vi "Testing Run.vi"(1 "FrequencyCounter":refnum<visa-resource-name>, 2 "connection information":path, 4 "Output Powers":bool, 5 "Warmup":bool, 6 "PHN Test":bool, 7 "System Number":string, 8 "error in":errorcluster, 9 "Osc Test":bool, 10 "FVT Test":bool, 11 "Arduino":refnum<visa-resource-name>) -> (0 "error out":errorcluster, 3 "Arduino out":refnum<visa-resource-name>)   [LabVIEW 2024]
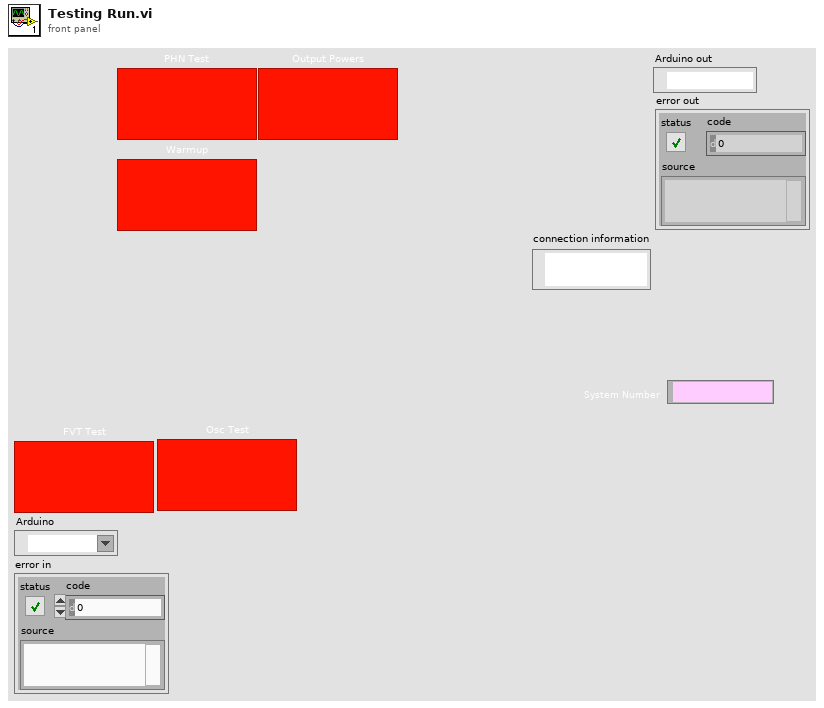
[diagram p1: front panel]
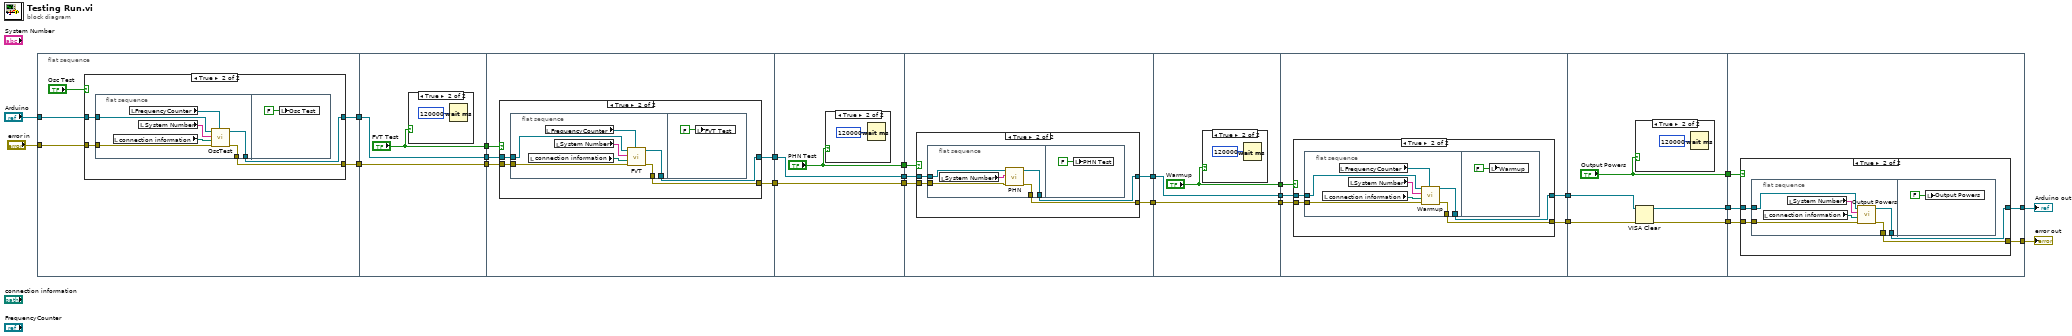
[diagram p0: block diagram]
diagram:
  n1 = flat-sequence {
    tunnel: [w26] -> w8
    tunnel: [w25] -> w6
    tunnel: "error in" -> [w28]
    tunnel: "Arduino" -> [w27]
    tunnel: w8 -> [w46]
    tunnel: [w46] -> w7
    tunnel: w6 -> [w45]
    tunnel: [w45] -> w5
    tunnel: ["FVT Test"] -> w4
    tunnel: w7 -> [w52]
    tunnel: w5 -> [w51]
    tunnel: [w50] -> w12
    tunnel: [w49] -> w10
    tunnel: w4 -> [w48]
    tunnel: w12 -> [w69]
    tunnel: [w69] -> w11
    tunnel: w10 -> [w68]
    tunnel: [w68] -> w9
    tunnel: ["PHN Test"] -> w3
    tunnel: w11 -> [w75]
    tunnel: w9 -> [w74]
    tunnel: [w73] -> w16
    tunnel: [w72] -> w14
    tunnel: w3 -> [w71]
    tunnel: w16 -> [w90]
    tunnel: [w90] -> w15
    tunnel: w14 -> [w89]
    tunnel: [w89] -> w13
    tunnel: ["Warmup"] -> w2
    tunnel: w15 -> [w96]
    tunnel: w13 -> [w94]
    tunnel: [w95] -> w20
    tunnel: [w93] -> w18
    tunnel: w2 -> [w92]
    tunnel: w20 -> [w115]
    tunnel: [w112] -> w19
    tunnel: w18 -> [w114]
    tunnel: [w113] -> w17
    tunnel: ["Output Powers"] -> w1
    tunnel: [w118] -> w21
    tunnel: [w120] -> w22
    tunnel: w19 -> [w121]
    tunnel: w17 -> [w119]
    tunnel: w1 -> [w117]
    frame #0 {
      n2 = case shown="True" "Osc Test" {
        tunnel: w28 -> [w30 w35]
        tunnel: w27 -> [w31 w34]
        tunnel: [w31 w33] -> w26
        tunnel: [w30 w32] -> w25
        frame False {
        }
        frame True {
          n3 = flat-sequence {
            tunnel: w35 -> [w41]
            tunnel: w34 -> [w40]
            tunnel: [w39] -> w33
            tunnel: [w38] -> w32
            frame #0 {
              n4 = local read "connection information"() -> (w37:path)
              n5 = local read "FrequencyCounter"() -> (w36:refnum<visa-resource-name>)
              n6 = local read "System Number"() -> (w42:string)
              n7 = call "OscTest.vi"("FrequencyCounter"=w36, "error in"=w41, "connection information"=w37, "System Number"=w42, "Arduino"=w40) -> ("error out"=w38:errorcluster, "Arduino out"=w39:refnum<visa-resource-name>)  [unwired: 5 in]
            }
            frame #1 {
              n8 = local write "Osc Test"(FALSE ("Osc Test")) -> ()
            }
          }
        }
      }
    }
    frame #1 {
      n9 = case shown="True" "FVT Test" {
        frame False {
        }
        frame True {
          n10 = Wait (ms)(milliseconds to wait=u32 120000) -> ()  [unwired: 1 out]
        }
      }
    }
    frame #2 {
      n11 = case shown="True" w48 {
        tunnel: w51 -> [w54 w57]
        tunnel: w52 -> [w53 w58]
        tunnel: [w53 w56] -> w50
        tunnel: [w54 w55] -> w49
        frame False {
        }
        frame True {
          n12 = flat-sequence {
            tunnel: w58 -> [w65]
            tunnel: w57 -> [w64]
            tunnel: [w62] -> w56
            tunnel: [w61] -> w55
            frame #0 {
              n13 = local read "connection information"() -> (w60:path)
              n14 = local read "FrequencyCounter"() -> (w59:refnum<visa-resource-name>)
              n15 = local read "System Number"() -> (w63:string)
              n16 = call "FVT.vi"("FrequencyCounter"=w59, "error in"=w64, "connection information"=w60, "System Number"=w63, "Arduino"=w65) -> ("error out"=w61:errorcluster, "Arduino out"=w62:refnum<visa-resource-name>)  [unwired: 5 in]
            }
            frame #1 {
              n17 = local write "FVT Test"(FALSE ("FVT Test")) -> ()
            }
          }
        }
      }
    }
    frame #3 {
      n18 = case shown="True" "PHN Test" {
        frame False {
        }
        frame True {
          n19 = Wait (ms)(milliseconds to wait=u32 120000) -> ()  [unwired: 1 out]
        }
      }
    }
    frame #4 {
      n20 = case shown="True" w71 {
        tunnel: w75 -> [w77 w81]
        tunnel: w74 -> [w76 w80]
        tunnel: [w77 w79] -> w73
        tunnel: [w76 w78] -> w72
        frame False {
        }
        frame True {
          n21 = flat-sequence {
            tunnel: w81 -> [w86]
            tunnel: w80 -> [w85]
            tunnel: [w84] -> w79
            tunnel: [w83] -> w78
            frame #0 {
              n22 = local read "System Number"() -> (w82:string)
              n23 = call "PHN.vi"("error in"=w85, "System Number"=w82, "Arduino"=w86) -> ("error out"=w83:errorcluster, "Arduino out"=w84:refnum<visa-resource-name>)  [unwired: 7 in]
            }
            frame #1 {
              n24 = local write "PHN Test"(FALSE ("PHN Test")) -> ()
            }
          }
        }
      }
    }
    frame #5 {
      n25 = case shown="True" "Warmup" {
        frame False {
        }
        frame True {
          n26 = Wait (ms)(milliseconds to wait=u32 120000) -> ()  [unwired: 1 out]
        }
      }
    }
    frame #6 {
      n27 = case shown="True" w92 {
        tunnel: w96 -> [w98 w102]
        tunnel: [w98 w101] -> w95
        tunnel: [w97 w99] -> w93
        tunnel: w94 -> [w97 w100]
        frame False {
        }
        frame True {
          n28 = flat-sequence {
            tunnel: w102 -> [w109]
            tunnel: [w108] -> w101
            tunnel: [w107] -> w99
            tunnel: w100 -> [w105]
            frame #0 {
              n29 = local read "connection information"() -> (w104:path)
              n30 = local read "FrequencyCounter"() -> (w103:refnum<visa-resource-name>)
              n31 = local read "System Number"() -> (w106:string)
              n32 = call "Warmup.vi"("FrequencyCounter"=w103, "error in"=w105, "connection information"=w104, "System Number"=w106, "Arduino in"=w109) -> ("error out"=w107:errorcluster, "Arduino out"=w108:refnum<visa-resource-name>)  [unwired: 5 in]
            }
            frame #1 {
              n33 = local write "Warmup"(FALSE ("PHN Test")) -> ()
            }
          }
        }
      }
    }
    frame #7 {
      n34 = case shown="True" "Output Powers" {
        frame False {
        }
        frame True {
          n35 = Wait (ms)(milliseconds to wait=u32 120000) -> ()  [unwired: 1 out]
        }
      }
      n36 = VISA Clear(VISA resource name=w115, error in (no error)=w114) -> (VISA resource name out=w112:refnum<visa-resource-name>, error out=w113:errorcluster)
    }
    frame #8 {
      n37 = case shown="True" w117 {
        tunnel: w121 -> [w123 w127]
        tunnel: [w123 w126] -> w120
        tunnel: w119 -> [w122 w125]
        tunnel: [w122 w124] -> w118
        frame False {
        }
        frame True {
          n38 = flat-sequence {
            tunnel: w125 -> [w129]
            tunnel: [w133] -> w126
            tunnel: [w132] -> w124
            tunnel: w127 -> [w130]
            frame #0 {
              n39 = local read "connection information"() -> (w128:path)
              n40 = local read "System Number"() -> (w131:string)
              n41 = call "Output Powers.vi"("error in"=w129, "connection information"=w128, "System Number"=w131, "Arduino in"=w130) -> ("error out"=w132:errorcluster, "Arduino out"=w133:refnum<visa-resource-name>)  [unwired: 6 in]
            }
            frame #1 {
              n42 = local write "Output Powers"(FALSE ("PHN Test")) -> ()
            }
          }
        }
      }
    }
  }
  "Arduino out" <- w22
  "error out" <- w21
